vi "Transmit Lockin Data.vi"(8 "error in (no error)":errorcluster, 9 "Reset":bool, 10 "Data":dbl[](array[numeric]), 11 "RP Transceiver in":refnum<class "RP Transceiver.lvclass">) -> (0 "error out":errorcluster, 2 "First phase word":i32, 3 "RP Transceiver out":refnum<class "RP Transceiver.lvclass">)   [LabVIEW 2016, in "RP Transceiver.lvclass"]
uses:
  RP Transceiver.lvclass
  RP Transceiver.lvclass/RP Transceiver.ctl
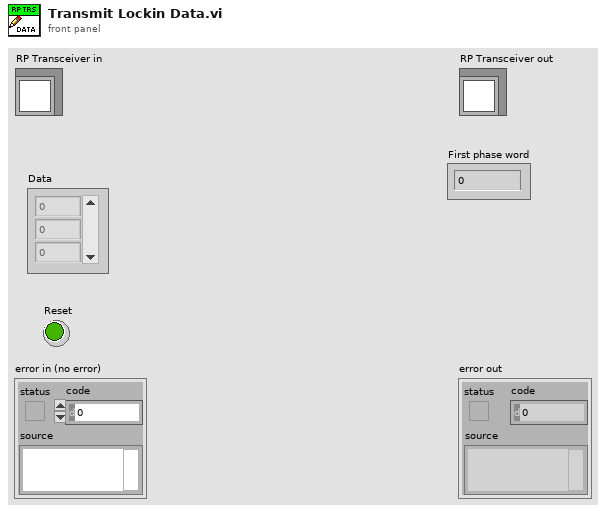
[diagram p1: front panel]
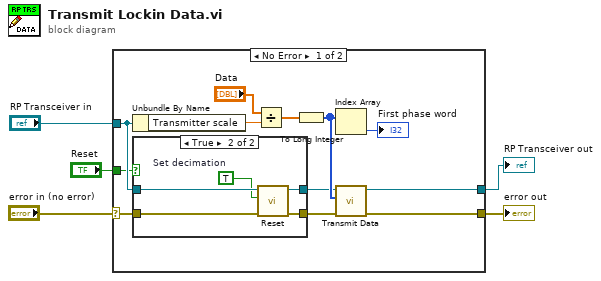
[diagram p0: block diagram]
diagram:
  n1 = case shown="No Error" "error in (no error)" {
    selector: "error in (no error)" -> [w13 w26]
    tunnel: [w12 w26] -> w4
    tunnel: [w17 w25] -> w2
    tunnel: "RP Transceiver in" -> [w7 w25]
    tunnel: "Reset" -> [w6 _]
    frame No Error {
      n2 = Unbundle By Name(w7) -> ("Transmitter scale"=w15:dbl)
      n3 = case shown="True" w6 {
        tunnel: w13 -> [w19 w24]
        tunnel: [w19 w23] -> w9
        tunnel: [w18 w22] -> w8
        tunnel: w7 -> [w18 w21]
        frame False {
        }
        frame True {
          w20 = TRUE  # Set decimation
          n4 = call-dynamic "Reset.vi"("error in (no error)"=w24, "Set decimation"=w20, "RP Instrument in"=w21) -> ("error out"=w23:errorcluster, "RP Instrument out"=w22:refnum<class "RP Transceiver.lvclass">)  [unwired: 7 in]
        }
      }
      n5 = Divide(x="Data", y=w15) -> (x/y=w14:dbl[])
      n6 = To Long Integer(number=w14) -> (32bit integer=w11:i32[])
      n7 = Index Array(array=w11) -> (element=→"First phase word":i32)  [unwired: 1 in]
      n8 = call-dynamic "Transmit Data.vi"("error in (no error)"=w9, "Data"=w11, "RP Instrument in"=w8) -> ("error out"=w12:errorcluster, "RP Instrument out"=w17:refnum<class "RP Transceiver.lvclass">)  [unwired: 7 in]
    }
    frame Error {
    }
  }
  "error out" <- w4
  "RP Transceiver out" <- w2
